vi "Land or Take Off(SubVI).vi"(10 "Land/Take off In":bool, 11 "Toggle Land/Take off":bool) -> (3 "Boolean":bool)   [LabVIEW 2014]
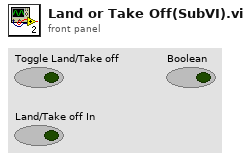
[diagram p1: front panel]
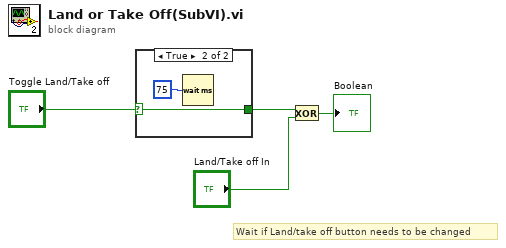
[diagram p0: block diagram]
diagram:
  # "Wait if Land/take off button needs to be changed"
  n1 = case shown="True" "Toggle Land/Take off" {
    selector: "Toggle Land/Take off" -> [w5 w7]
    tunnel: [w5 w7] -> w1
    frame False {
    }
    frame True {
      n2 = Wait (ms)(milliseconds to wait=u32 75) -> ()  [unwired: 1 out]
    }
  }
  n3 = Exclusive Or(1:"Land/Take off In", 2:w1) -> (0:→"Boolean":bool)
